vi "Request Data JSON.vi"(8 "error in (no error)":errorcluster, 11 "SetPersistentData in":refnum<class "SetPersistentData.lvclass">) -> (0 "error out":errorcluster, 2 "Request Data JSON":string, 3 "SetPersistentData out":refnum<class "SetPersistentData.lvclass">)   [LabVIEW 2022 SP3, in "obs-websocket-lv.lvlib" / "SetPersistentData.lvclass"]
uses:
  SetPersistentData.lvclass
  SetPersistentData.lvclass/SetPersistentData.ctl
  <vilib>/IlluminatedG/lv-web-crypto/lv-json/JSON/JSON.lvlib
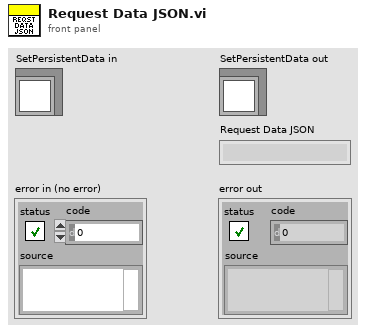
[diagram p1: front panel]
types:
  T1 = typedef "obs-websocket-lv.lvlib/Data Realm.ctl" = enum16{"Global", "Profile"}
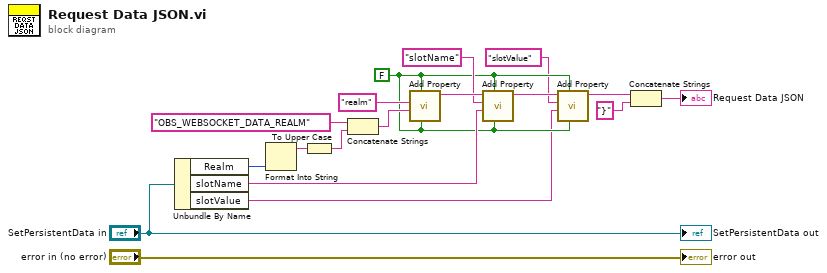
[diagram p0: block diagram]
diagram:
  w5 = FALSE ("Include Empty?")
  n1 = Unbundle By Name("SetPersistentData in") -> ("Realm"=w17:T1, "slotName"=w9:string, "slotValue"=w3:string)
  n2 = Format Into String(w17) -> (resulting string=w16:string)  [unwired: 3 in, 1 out]
  n3 = To Upper Case(1:w16) -> (0:w15:string)
  n4 = Concatenate Strings("OBS_WEBSOCKET_DATA_REALM" ("string"), w15) -> (w12:string)
  n5 = call <vilib>:"Add Property.vi"("String?"=w5, "Include Empty?"=w5, "Value"=w12, "Property Name"="realm") -> ("String out"=w11:string)  [unwired: 7 in]
  n6 = call <vilib>:"Add Property.vi"("String?"=w5, "Include Empty?"=w5, "Value"=w9, "Property Name"="slotName", "String In"=w11) -> ("String out"=w6:string)  [unwired: 6 in]
  n7 = call <vilib>:"Add Property.vi"("String?"=w5, "Include Empty?"=w5, "Value"=w3, "Property Name"="slotValue", "String In"=w6) -> ("String out"=w2:string)  [unwired: 6 in]
  n8 = Concatenate Strings(w2, "}" ("string")) -> (→"Request Data JSON":string)
  "error out" <- "error in (no error)"
  "SetPersistentData out" <- "SetPersistentData in"
